vi "Global_HW_Address_FINAL_Assignments.vi"() -> ()   [LabVIEW 2017]
uses:
  <vilib>/Rock Robotics/WPI/Joystick/WPI_JoystickDeviceEnum.ctl
  <vilib>/Rock Robotics/SystemInterfaces/DIO/FPGA_DIOChannel.ctl
  <vilib>/Rock Robotics/WPI/SerialPort/WPI_SerialPort.ctl
  <vilib>/Rock Robotics/WPI/ThirdParty/CanMotor/TalonSRX/WPI_CANTalonSRX_BrakeOverride.ctl
  <vilib>/Rock Robotics/SystemInterfaces/AI/FPGA_AIChannel.ctl
  <vilib>/Rock Robotics/SystemInterfaces/DIO/FPGA_DIOPWMChannel.ctl
panel:
  in  "GEAR Servo Left":T1
  in  "GEAR Servo Right":T1=enum."PWM 1"
  in  "Sonar Scaling Factor":dbl=0.0235
  in  "Sonar Average Bits":u8
  in  "Sonar Channel":T2=enum."AI 3"
  in  "Shooter Wheel":T4={"Shooter Wheel Motor"=17, "Invert Wheel Motor"=FALSE, "Reverse Wheel Feedback Sensor"=FALSE, "Forward Peak Output"=0.0, "Reverse Peak Output"=-1.0, "Brake / Coast Mode"=enum."Override to Coast"}
  in  "Shooter Hood":T5={"Shooter Hood Motor"=3, "Invert Hood Motor"=FALSE, "Reverse Hood Feedback Sensor"=FALSE, "Forward Limit Position"=23.0, "Reverse Limit Position"=0.0}
  in  "Mechamon Drive":T6={"Rear Left Motor "=15, "Invert Rear Left"=TRUE, "Rear Right Motor"=11, "Invert Rear Right"=FALSE, "Front Left Motor"=0, "Invert Front Left"=TRUE, "Front Right Motor"=0, "Invert Front Right"=FALSE}
  in  "Arduino Port":T8={"Serial Port"=enum."Onboard RS-232", "Baud Rate"=115200, "Data Bits"=8, "Parity"=0, "Stop Bits"=10, "Flow Control"=0} {"Flow Control" items=["None", "XON/XOFF", "RTS/CTS", "XON/XOFF & RTS/CTS", "DTR/DSR", "XON/XOFF & DTR/DSR"]; "Stop Bits" items=["1.0"=10, "1.5"=15, "2.0"=20]; "Parity" items=["None", "Odd", "Even", "Mark", "Space"]}
  in  "Intake Motor":u8=12
  in  "Ball Agitator Motor":u8=9
  in  "Hopper Sensor":T9=enum."DIO 1"
  in  "Ball Feeder Motor":u8=14
  in  "Gear Sensor":T9
  in  "Button Board":T10=enum."USB 1"
  in  "Joystick":T10
  out "Invert Climber Motor":bool
  in  "Climber Motor":u8=1
  # "#HW_Adress\nAssign Motor Addresses\nWhen Given\nAssign in Global_HW_Address_Assignment.vi"
  # "#HW_Assigments These globals are used to assign\nthe HW settings for the robot. HW state machines should\nuse these global variables to ease updates if any HW\nchanges have been made."
  # "Sonar"
  # "Intake"
  # "Hopper System"
  # "Gear System"
  # "Controllers"
  # "Climber"
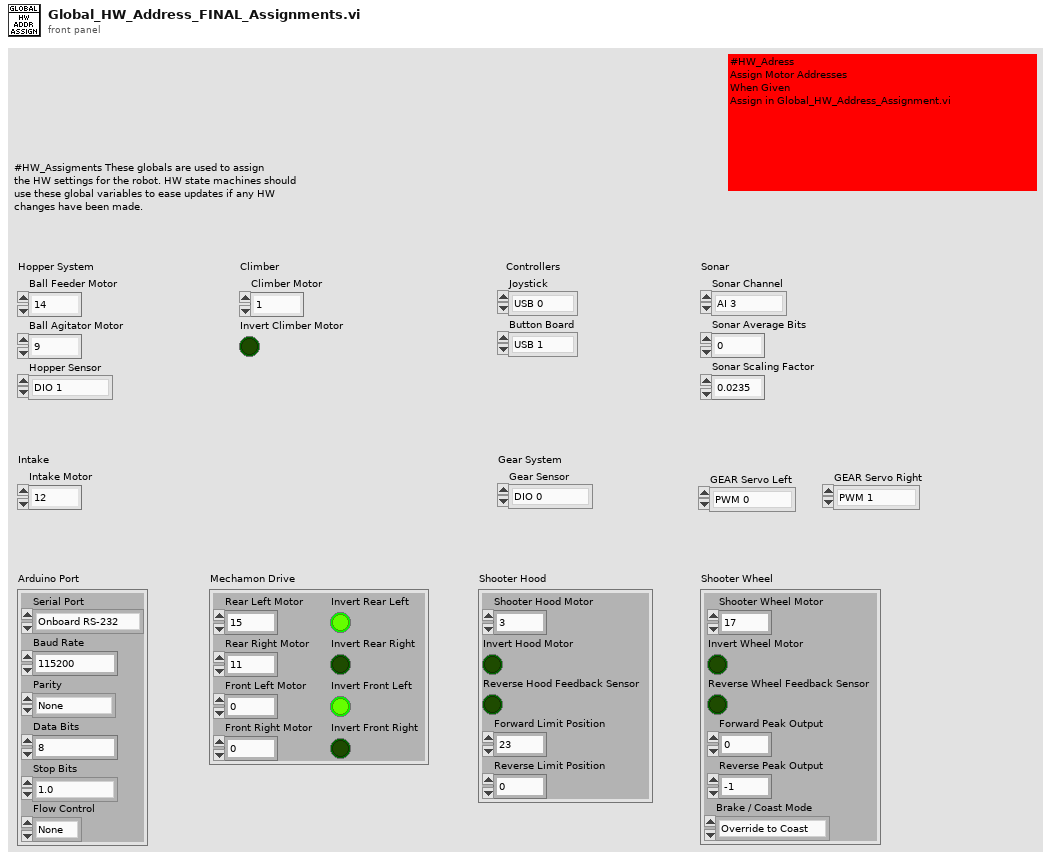
[diagram p1: front panel]
types:
  T1 = typedef "FPGA_DIOPWMChannel.ctl" = enum8{"PWM 0", "PWM 1", "PWM 2", "PWM 3", "PWM 4", "PWM 5", "PWM 6", "PWM 7", "PWM 8", "PWM 9", "PWM MXP 0", "PWM MXP 1", "PWM MXP 2", "PWM MXP 3", "PWM MXP 4", "PWM MXP 5", "PWM MXP 6", "PWM MXP 7", "PWM MXP 8", "PWM MXP 9", "Invalid"}
  T2 = typedef "FPGA_AIChannel.ctl" = enum8{"AI 0", "AI 1", "AI 2", "AI 3", "AI MXP 0", "AI MXP 1", "AI MXP 2", "AI MXP 3", "Invalid"}
  T3 = typedef "WPI_CANTalonSRX_BrakeOverride.ctl" = enum8{"No Override", "Override to Coast", "Override to Brake"}
  T4 = cluster{"Shooter Wheel Motor":u8, "Invert Wheel Motor":bool, "Reverse Wheel Feedback Sensor":bool, "Forward Peak Output":dbl, "Reverse Peak Output":dbl, "Brake / Coast Mode":T3}
  T5 = cluster{"Shooter Hood Motor":u8, "Invert Hood Motor":bool, "Reverse Hood Feedback Sensor":bool, "Forward Limit Position":dbl, "Reverse Limit Position":dbl}
  T6 = cluster{"Rear Left Motor ":u8, "Invert Rear Left":bool, "Rear Right Motor":u8, "Invert Rear Right":bool, "Front Left Motor":u8, "Invert Front Left":bool, "Front Right Motor":u8, "Invert Front Right":bool}
  T7 = typedef "WPI_SerialPort.ctl" = enum16{"Onboard RS-232", "MXP TTL", "USB 1", "USB 2"}
  T8 = cluster{"Serial Port":T7, "Baud Rate":u32, "Data Bits":u16, "Parity":u16, "Stop Bits":u16, "Flow Control":u16}
  T9 = typedef "FPGA_DIOChannel.ctl" = enum8{"DIO 0", "DIO 1", "DIO 2", "DIO 3", "DIO 4", "DIO 5", "DIO 6", "DIO 7", "DIO 8", "DIO 9", "DIO MXP 0", "DIO MXP 1", "DIO MXP 2", "DIO MXP 3", "DIO MXP 4", "DIO MXP 5", "DIO MXP 6", "DIO MXP 7", "DIO MXP 8", "DIO MXP 9", "DIO MXP 10", "DIO MXP 11", "DIO MXP 12", "DIO MXP 13", "DIO MXP 14", "DIO MXP 15", "SPI Port CS1", "SPI Port CS2", "SPI Port CS3", "SPI Port MISO", "SPI Port MOSI", "Invalid"}
  T10 = typedef "WPI_JoystickDeviceEnum.ctl" = enum16{"USB 0", "USB 1", "USB 2", "USB 3", "USB 4", "USB 5"}
diagram:
